vi "Set Count Behaviour.vi"(8 "error in (no error)":errorcluster, 10 "Count Behaviour":T1) -> (0 "error out":errorcluster)   [LabVIEW 2020, in "Test Actor API.lvclass"]
uses:
  Test Actor API.lvclass
  Actor/Count Behaviour.ctl
  Base Actor/API/Actor API.lvclass/Actor API.ctl
  Base Actor/API/Actor API.lvclass
  Global Framework References.vi
  C:/dev/PGS/2001 - TBCM/Source/RT/RTAF/Source/RTAF/Actors/Base Actor/API/Actor API.lvclass
  C:/dev/PGS/2001 - TBCM/Source/RT/RTAF/Source/RTAF/Actors/Test/API/Test Actor API.lvclass
  Actor/Test Actor.lvclass
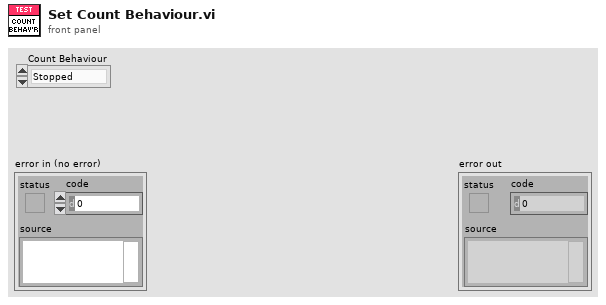
[diagram p1: front panel]
types:
  T1 = typedef "Test Actor.lvclass/Count Behaviour.ctl" = enum16{"Stopped", "Up", "Down"}
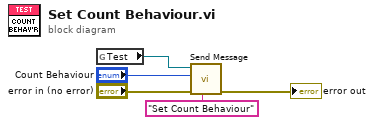
[diagram p0: block diagram]
diagram:
  n1 = global read "Global Framework References.vi" "Test"() -> (w1:refnum<class "Test Actor API.lvclass">)
  n2 = call "Send Message.vi"("Name"="Set Count Behaviour", "error in (no error)"="error in (no error)", "Payload"="Count Behaviour", "Actor API in"=w1) -> ("error out"=→"error out":errorcluster)  [unwired: 7 in]
